vi "AppPath.vi"(8 "error in (no error)":errorcluster) -> (0 "error out":errorcluster, 2 "App Folder":path)   [LabVIEW 2020]
uses:
  <vilib>/Utility/sysdir.llb/System Directory Type.ctl
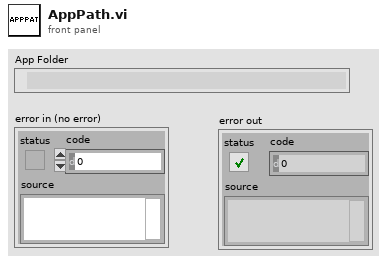
[diagram p1: front panel]
types:
  T1 = enum16{"open", "replace", "create", "open or create", "replace or create", "replace or create with confirmation"}
  T2 = typedef "System Directory Type.ctl" = i32
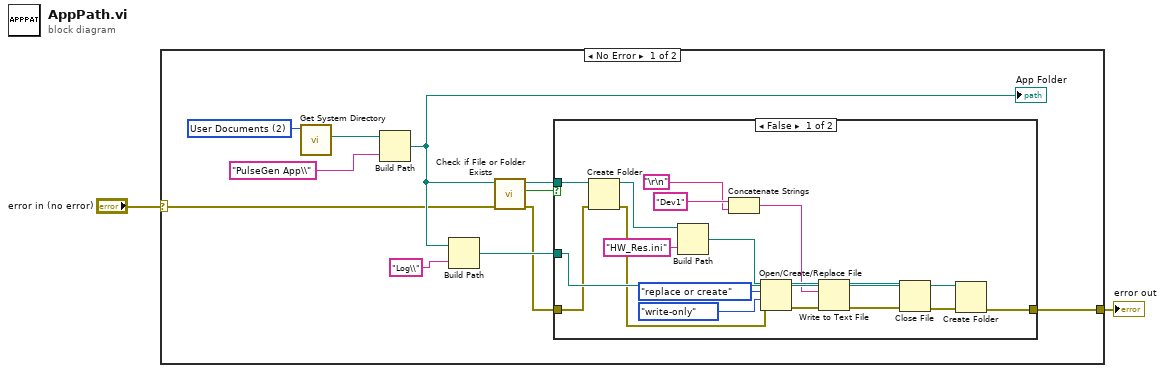
[diagram p0: block diagram]
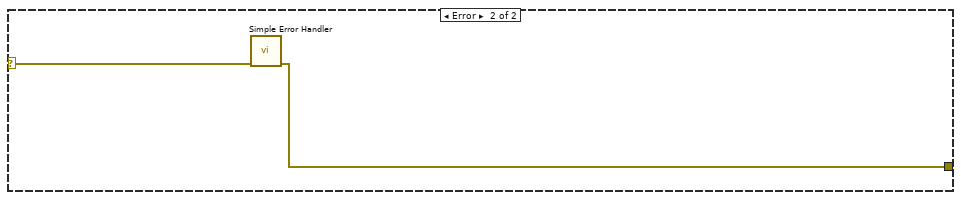
[diagram p3: hidden frame]
diagram:
  n1 = case shown="No Error" "error in (no error)" {
    selector: "error in (no error)" -> [w4 w34]
    tunnel: [w3 w33] -> w1
    frame No Error {
      w7 = T2 2 items=["User Home", "User Desktop", "User Documents", "User Application Data", "User Preferences", "User Temporary", "Public Documents", "Public Application Data", "Public Preferences", "System Core Libraries", "System Installed Libraries", "Application Files", "Boot Volume Root"] ("system directory type")
      n2 = call <vilib>:"Get System Directory.vi"("system directory type"=w7) -> ("system directory"=w8:path)  [unwired: 10 in]
      n3 = Build Path(base path=w8, name or relative path="PulseGen App\\") -> (appended path=w5:path)
      "App Folder" <- w5
      n4 = Build Path(base path=w5, name or relative path="Log\\") -> (appended path=w13:path)
      n5 = call <vilib>:"Check if File or Folder Exists.vi"("error in (no error)"=w4, "path"=w5) -> ("error out"=w6:errorcluster, "file or folder exists?"=w10:bool, "dup path"=w11:path)  [unwired: 7 in]
      n6 = case shown="False" w10 {
        tunnel: w11 -> [w31 _]
        tunnel: w13 -> [w30 _]
        tunnel: w6 -> [w16 w32]
        tunnel: [w29 w32] -> w3
        frame False {
          n7 = Create Folder(path (use dialog)=w31, error in=w16) -> (created path=w15:path, error out=w14:errorcluster)  [unwired: 1 in, 1 out]
          n8 = Build Path(base path=w15, name or relative path="HW_Res.ini") -> (appended path=w28:path)
          n9 = Concatenate Strings("Dev1" ("string"), "\r\n") -> (w25:string)
          n10 = Open/Create/Replace File(file path (use dialog)=w28, error in=w14, operation (0:open)=T1."replace or create", access (0:read/write)=enum16{"read/write", "read-only", "write-only"}."write-only") -> (refnum out=w26:refnum<file>, error out=w27:errorcluster)  [unwired: 2 in, 1 out]
          n11 = Write to Text File(file (use dialog)=w26, text=w25, error in=w27) -> (refnum out=w23:refnum<file>, error out=w24:errorcluster)  [unwired: 1 in, 1 out]
          n12 = Close File(refnum=w23, error in=w24) -> (error out=w17:errorcluster)  [unwired: 1 out]
          n13 = Create Folder(path (use dialog)=w30, error in=w17) -> (error out=w29:errorcluster)  [unwired: 1 in, 2 out]
        }
        frame True {
        }
      }
    }
    frame Error {
      n14 = call <vilib>:"Simple Error Handler.vi"("error in (no error)"=w34) -> ("error out"=w33:errorcluster)  [unwired: 4 in, 4 out]
    }
  }
  "error out" <- w1
